vi "User data_Cnsl.vi"(0 "Inspector":string="ID-0", 1 "base path":path=path "C:/", 2 "prompt (Create Folder)":string="logsConsole", 5 "Station":string="EQD", 7 "Vendor":string="Icon", 9 "Number":string="?", 11 "Error In":errorcluster, 12 "file name":string, 13 "PO#":string="?") -> (4 "refnum out":refnum<file>, 15 "error out":errorcluster)   [LabVIEW 2018]
uses:
  Global_usbComm.vi
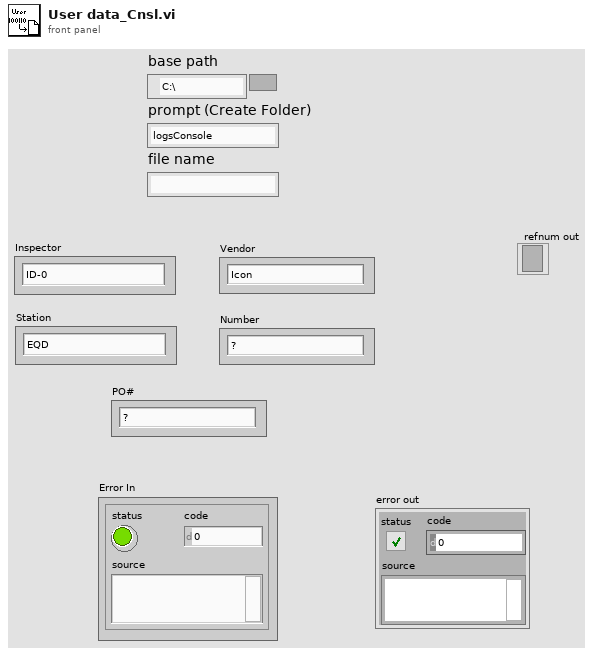
[diagram p1: front panel]
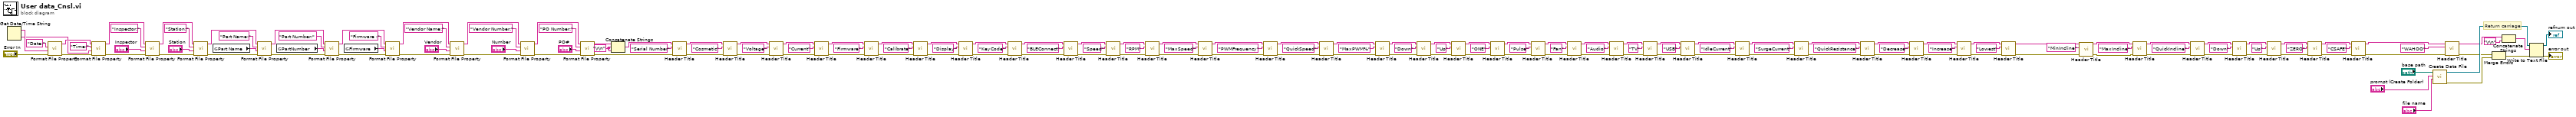
[diagram p0: block diagram]
diagram:
  w128 = "\r\n"
  # "Return carriage"
  n1 = Get Date/Time String() -> (date string=w7:string, time string=w6:string)  [unwired: 3 in]
  n2 = call "Format File Property.vi"("Error In"="Error In", "File Property Value"=w7, "File Property Name"="Date:") -> ("Error Out"=w160:errorcluster, "String out"=w97:string)  [unwired: 7 in]
  n3 = call "Format File Property.vi"("Error In"=w160, "File Property Value"=w6, "File Property Name"="Time:", "String in"=w97) -> ("Error Out"=w161:errorcluster, "String out"=w96:string)  [unwired: 6 in]
  n4 = call "Format File Property.vi"("Error In"=w161, "File Property Value"="Inspector", "File Property Name"="Inspector:", "String in"=w96) -> ("Error Out"=w159:errorcluster, "String out"=w95:string)  [unwired: 6 in]
  n5 = call "Format File Property.vi"("Error In"=w159, "File Property Value"="Station", "File Property Name"="Station:", "String in"=w95) -> ("Error Out"=w153:errorcluster, "String out"=w94:string)  [unwired: 6 in]
  n6 = global read "Global_usbComm.vi" "Part Name"() -> (w81:string)
  n7 = call "Format File Property.vi"("Error In"=w153, "File Property Value"=w81, "File Property Name"="Part Name:", "String in"=w94) -> ("Error Out"=w152:errorcluster, "String out"=w93:string)  [unwired: 6 in]
  n8 = global read "Global_usbComm.vi" "PartNumber"() -> (w80:string)
  n9 = call "Format File Property.vi"("Error In"=w152, "File Property Value"=w80, "File Property Name"="Part Number:", "String in"=w93) -> ("Error Out"=w162:errorcluster, "String out"=w92:string)  [unwired: 6 in]
  n10 = global read "Global_usbComm.vi" "Firmware"() -> (w79:string)
  n11 = call "Format File Property.vi"("Error In"=w162, "File Property Value"=w79, "File Property Name"="Firmware :", "String in"=w92) -> ("Error Out"=w163:errorcluster, "String out"=w91:string)  [unwired: 6 in]
  n12 = call "Format File Property.vi"("Error In"=w163, "File Property Value"="Vendor", "File Property Name"="Vendor Name:", "String in"=w91) -> ("Error Out"=w164:errorcluster, "String out"=w90:string)  [unwired: 6 in]
  n13 = call "Format File Property.vi"("Error In"=w164, "File Property Value"="Number", "File Property Name"="Vendor Number:", "String in"=w90) -> ("Error Out"=w10:errorcluster, "String out"=w11:string)  [unwired: 6 in]
  n14 = call "Format File Property.vi"("Error In"=w10, "File Property Value"="PO#", "File Property Name"="PO Number:", "String in"=w11) -> ("Error Out"=w8:errorcluster, "String out"=w9:string)  [unwired: 6 in]
  n15 = Concatenate Strings(w9, w128, w128) -> (w129:string)
  n16 = call "Header Title.vi"("Error In"=w8, "Header Title"="Serial Number" ("string"), "String in"=w129) -> ("Error Out"=w101:errorcluster, "String out"=w100:string)  [unwired: 7 in]
  n17 = call "Header Title.vi"("Error In"=w101, "Header Title"="Cosmetic", "String in"=w100) -> ("Error Out"=w105:errorcluster, "String out"=w104:string)  [unwired: 7 in]
  n18 = call "Header Title.vi"("Error In"=w105, "Header Title"="Voltage", "String in"=w104) -> ("Error Out"=w98:errorcluster, "String out"=w99:string)  [unwired: 7 in]
  n19 = call "Header Title.vi"("Error In"=w98, "Header Title"="Current" ("string"), "String in"=w99) -> ("Error Out"=w58:errorcluster, "String out"=w59:string)  [unwired: 7 in]
  n20 = call "Header Title.vi"("Error In"=w58, "Header Title"="Firmware" ("string"), "String in"=w59) -> ("Error Out"=w57:errorcluster, "String out"=w56:string)  [unwired: 7 in]
  n21 = call "Header Title.vi"("Error In"=w57, "Header Title"="Calibrate" ("string"), "String in"=w56) -> ("Error Out"=w110:errorcluster, "String out"=w133:string)  [unwired: 7 in]
  n22 = call "Header Title.vi"("Error In"=w110, "Header Title"="Display" ("string"), "String in"=w133) -> ("Error Out"=w33:errorcluster, "String out"=w32:string)  [unwired: 7 in]
  n23 = call "Header Title.vi"("Error In"=w33, "Header Title"="KeyCode", "String in"=w32) -> ("Error Out"=w34:errorcluster, "String out"=w31:string)  [unwired: 7 in]
  n24 = call "Header Title.vi"("Error In"=w34, "Header Title"="BLEConnect", "String in"=w31) -> ("Error Out"=w21:errorcluster, "String out"=w20:string)  [unwired: 7 in]
  n25 = call "Header Title.vi"("Error In"=w21, "Header Title"="Speed", "String in"=w20) -> ("Error Out"=w19:errorcluster, "String out"=w18:string)  [unwired: 7 in]
  n26 = call "Header Title.vi"("Error In"=w19, "Header Title"="RPM", "String in"=w18) -> ("Error Out"=w16:errorcluster, "String out"=w17:string)  [unwired: 7 in]
  n27 = call "Header Title.vi"("Error In"=w16, "Header Title"="MaxSpeed", "String in"=w17) -> ("Error Out"=w123:errorcluster, "String out"=w126:string)  [unwired: 7 in]
  n28 = call "Header Title.vi"("Error In"=w123, "Header Title"="PWMFrequency", "String in"=w126) -> ("Error Out"=w83:errorcluster, "String out"=w84:string)  [unwired: 7 in]
  n29 = call "Header Title.vi"("Error In"=w83, "Header Title"="QuickSpeed", "String in"=w84) -> ("Error Out"=w48:errorcluster, "String out"=w49:string)  [unwired: 7 in]
  n30 = call "Header Title.vi"("Error In"=w48, "Header Title"="MaxPWM%" ("Measured Data"), "String in"=w49) -> ("Error Out"=w109:errorcluster, "String out"=w132:string)  [unwired: 7 in]
  n31 = call "Header Title.vi"("Error In"=w109, "Header Title"="Down" ("Measured Data"), "String in"=w132) -> ("Error Out"=w106:errorcluster, "String out"=w107:string)  [unwired: 7 in]
  n32 = call "Header Title.vi"("Error In"=w106, "Header Title"="Up", "String in"=w107) -> ("Error Out"=w124:errorcluster, "String out"=w127:string)  [unwired: 7 in]
  n33 = call "Header Title.vi"("Error In"=w124, "Header Title"="ONE", "String in"=w127) -> ("Error Out"=w46:errorcluster, "String out"=w47:string)  [unwired: 7 in]
  n34 = call "Header Title.vi"("Error In"=w46, "Header Title"="Pulse", "String in"=w47) -> ("Error Out"=w122:errorcluster, "String out"=w125:string)  [unwired: 7 in]
  n35 = call "Header Title.vi"("Error In"=w122, "Header Title"="Fan", "String in"=w125) -> ("Error Out"=w85:errorcluster, "String out"=w86:string)  [unwired: 7 in]
  n36 = call "Header Title.vi"("Error In"=w85, "Header Title"="Audio", "String in"=w86) -> ("Error Out"=w88:errorcluster, "String out"=w89:string)  [unwired: 7 in]
  n37 = call "Header Title.vi"("Error In"=w88, "Header Title"="TV", "String in"=w89) -> ("Error Out"=w114:errorcluster, "String out"=w115:string)  [unwired: 7 in]
  n38 = call "Header Title.vi"("Error In"=w114, "Header Title"="USB", "String in"=w115) -> ("Error Out"=w53:errorcluster, "String out"=w52:string)  [unwired: 7 in]
  n39 = call "Header Title.vi"("Error In"=w53, "Header Title"="IdleCurrent" ("Measured Data"), "String in"=w52) -> ("Error Out"=w25:errorcluster, "String out"=w26:string)  [unwired: 7 in]
  n40 = call "Header Title.vi"("Error In"=w25, "Header Title"="SurgeCurrent", "String in"=w26) -> ("Error Out"=w24:errorcluster, "String out"=w23:string)  [unwired: 7 in]
  n41 = call "Header Title.vi"("Error In"=w24, "Header Title"="QuickResistance", "String in"=w23) -> ("Error Out"=w63:errorcluster, "String out"=w64:string)  [unwired: 7 in]
  n42 = call "Header Title.vi"("Error In"=w63, "Header Title"="Decrease", "String in"=w64) -> ("Error Out"=w50:errorcluster, "String out"=w51:string)  [unwired: 7 in]
  n43 = call "Header Title.vi"("Error In"=w50, "Header Title"="Increase" ("Measured Data"), "String in"=w51) -> ("Error Out"=w27:errorcluster, "String out"=w28:string)  [unwired: 7 in]
  n44 = call "Header Title.vi"("Error In"=w27, "Header Title"="Lowest", "String in"=w28) -> ("Error Out"=w2:errorcluster, "String out"=w3:string)  [unwired: 7 in]
  n45 = call "Header Title.vi"("Error In"=w2, "Header Title"="MinIncline", "String in"=w3) -> ("Error Out"=w5:errorcluster, "String out"=w4:string)  [unwired: 7 in]
  n46 = call "Header Title.vi"("Error In"=w5, "Header Title"="MaxIncline", "String in"=w4) -> ("Error Out"=w37:errorcluster, "String out"=w38:string)  [unwired: 7 in]
  n47 = call "Header Title.vi"("Error In"=w37, "Header Title"="QuickIncline" ("Measured Data"), "String in"=w38) -> ("Error Out"=w45:errorcluster, "String out"=w44:string)  [unwired: 7 in]
  n48 = call "Header Title.vi"("Error In"=w45, "Header Title"="Down", "String in"=w44) -> ("Error Out"=w41:errorcluster, "String out"=w40:string)  [unwired: 7 in]
  n49 = call "Header Title.vi"("Error In"=w41, "Header Title"="Up", "String in"=w40) -> ("Error Out"=w35:errorcluster, "String out"=w36:string)  [unwired: 7 in]
  n50 = call "Header Title.vi"("Error In"=w35, "Header Title"="ZERO", "String in"=w36) -> ("Error Out"=w54:errorcluster, "String out"=w55:string)  [unwired: 7 in]
  n51 = call "Header Title.vi"("Error In"=w54, "Header Title"="CSAFE", "String in"=w55) -> ("Error Out"=w76:errorcluster, "String out"=w74:string)  [unwired: 7 in]
  n52 = call "Create Data File.vi"("file name"="file name", "prompt (Create Folder)"="prompt (Create Folder)", "base path"="base path") -> ("Error Out"=w154:errorcluster, "File Refnum"=w156:refnum<file>)  [unwired: 7 in]
  n53 = call "Header Title.vi"("Error In"=w76, "Header Title"="WAHOO", "String in"=w74) -> ("Error Out"=w75:errorcluster, "String out"=w73:string)  [unwired: 7 in]
  n54 = Merge Errors(w75, w154) -> (w155:errorcluster)
  n55 = Concatenate Strings(w73, "\r\n") -> (w130:string)
  n56 = Write to Text File(file (use dialog)=w156, text=w130, error in=w155) -> (refnum out=→"refnum out":refnum<file>, error out=→"error out":errorcluster)  [unwired: 1 in, 1 out]
